vi "Handle Messages.vi"(8 "error in (no error)":errorcluster, 9 "Message Data":variant, 10 "Message":string, 11 "Process In":refnum<class "Debugger.lvclass">) -> (0 "error out":errorcluster, 3 "Process Out":refnum<class "Debugger.lvclass">)   [LabVIEW 2020, in "Debugger.lvclass"]
doc: "This is the core VI handling incomming messages to the process. This VI should be overridden to add functionality to the process or override functionality implemented by a parent. Any message not handled should be sent to the parent method using the default case. \nEach state should be atomic and states should in general avoid enqueueing new messages from within this method, as there might be other messages interleaved in the queue from the outside. For cyclic iteration of an action, using a Helper Loop is recommended."
uses:
  Debugger.lvclass
  C:/Users/anton/Documents/GitHub/triarc-debugger/source/Process/Debug Process.lvclass
  Debug Data/Debug Data.lvclass
  Debugger.lvclass/Debugger.ctl
  Debug Log/Debug Log.lvclass/Debug Log.ctl
  Process/Debug Process.lvclass/Debug Process.ctl
  State Analyzer/Debug State Analyzer.lvclass/Debug State Analyzer.ctl
  Process/Public/Lifecycle/Get Lifecycle State.vi
  <vilib>/Utility/error.llb/Clear Errors.vi
  <vilib>/Utility/error.llb/Error Cluster From Error Code.vi
  Process/Debug Process.lvclass
  Filter/Filter.lvclass
  Debug Log/Debug Log.lvclass
  State Analyzer/Debug State Analyzer.lvclass
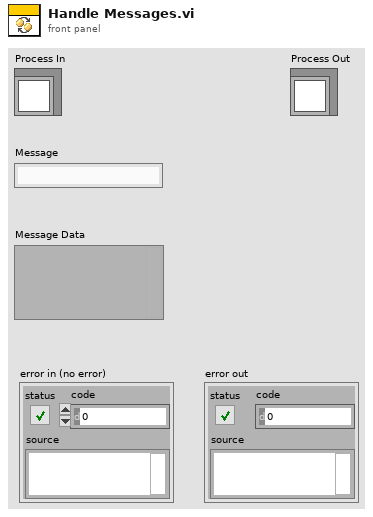
[diagram p1: front panel]
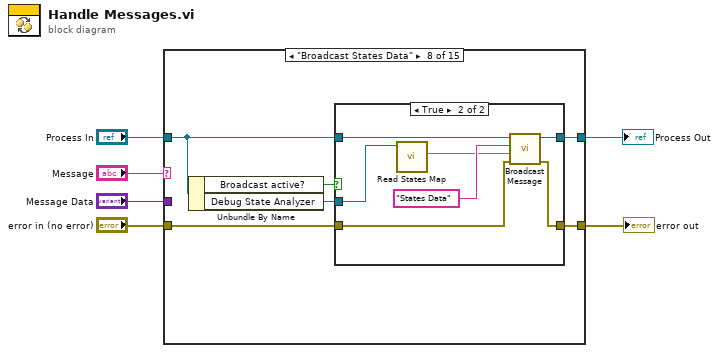
[diagram p0: block diagram]
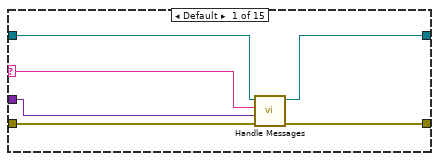
[diagram p2: hidden frame]
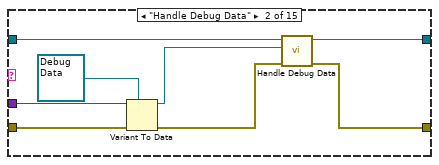
[diagram p3: hidden frame]
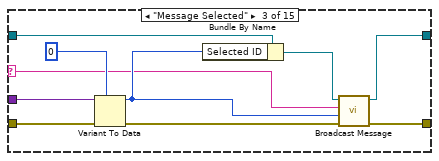
[diagram p4: hidden frame]
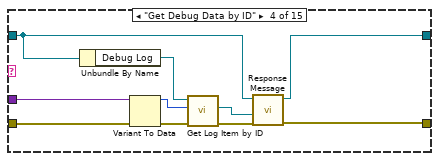
[diagram p5: hidden frame]
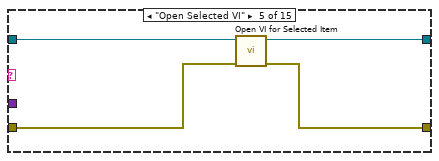
[diagram p6: hidden frame]
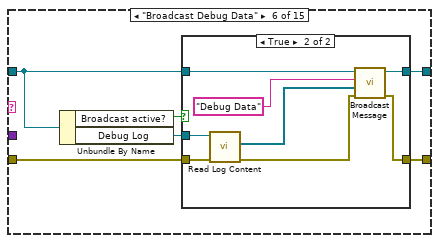
[diagram p7: hidden frame]
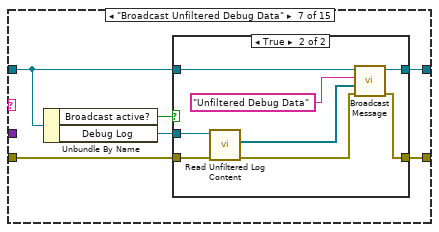
[diagram p9: hidden frame]
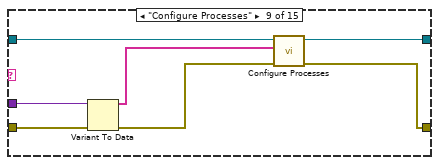
[diagram p12: hidden frame]
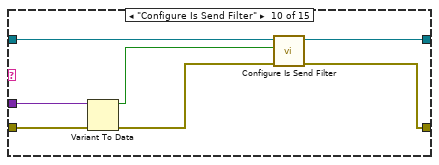
[diagram p13: hidden frame]
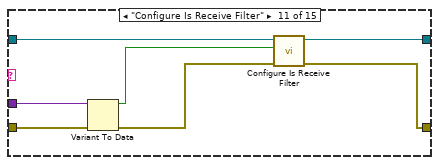
[diagram p14: hidden frame]
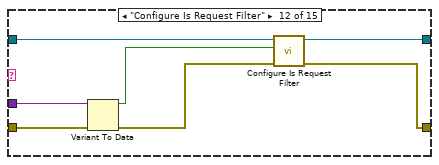
[diagram p15: hidden frame]
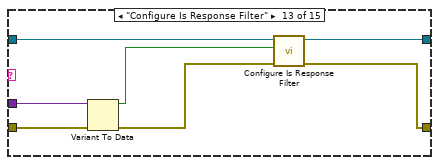
[diagram p16: hidden frame]
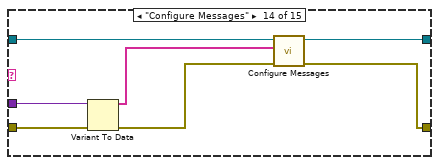
[diagram p17: hidden frame]
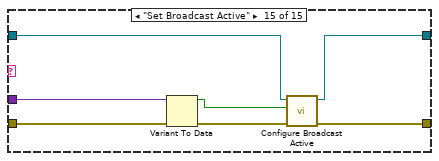
[diagram p18: hidden frame]
diagram:
  n1 = case shown="\"Broadcast States Data\"" "Message" {
    selector: "Message" -> [w8 _ w22 _ _ _ _ _ _ _ _ _ _ _ _]
    tunnel: [w12 w13 w25 w39 w41 w49 w65 w81 w93 w100 w107 w114 w121 w128 w137] -> w6
    tunnel: [w11 w15 w21 w40 w43 w50 w66 w82 w94 w101 w108 w115 w122 w129 w134] -> w5
    tunnel: "error in (no error)" -> [w10 w19 w29 w36 w44 w46 w62 w78 w98 w105 w112 w119 w126 w133 w139]
    tunnel: "Message Data" -> [w9 w20 w30 w37 _ _ _ _ w97 w104 w111 w118 w125 w132 w140]
    tunnel: "Process In" -> [w7 w16 w27 w32 w42 w48 w64 w80 w95 w102 w109 w116 w123 w130 w136]
    frame Default {
      n2 = call-parent "Handle Messages.vi"("error in (no error)"=w10, "Message Data"=w9, "Message"=w8, "Process In"=w7) -> ("error out"=w12:errorcluster, "Process Out"=w11:refnum<class "Debugger.lvclass">)  [unwired: 6 in]
    }
    frame "Handle Debug Data" {
      n3 = Variant To Data(error in=w19, type=refnum<class "Debug Data.lvclass"> refnum ("Debug Data.lvclass"), Variant=w20) -> (data=w14:refnum<class "Debug Data.lvclass">, error out=w17:errorcluster)
      n4 = call-dynamic "Handle Debug Data.vi"("error in (no error)"=w17, "Debug Data.lvclass"=w14, "Debug Data Event In"=w16) -> ("error out"=w13:errorcluster, "Debug Data Event Out"=w15:refnum<class "Debugger.lvclass">)  [unwired: 7 in]
    }
    frame "Message Selected" {
      n5 = Variant To Data(error in=w29, type=u32 0 ("Message ID"), Variant=w30) -> (data=w23:u32, error out=w26:errorcluster)
      n6 = Bundle By Name(cluster=w27, "Selected ID"=w23) -> (w24:refnum<class "Debugger.lvclass">)
      n7 = call-dynamic "Broadcast Message.vi"("error in (no error)"=w26, "Message Data"=w23, "Message"=w22, "Process In"=w24) -> ("error out"=w25:errorcluster, "Process Out"=w21:refnum<class "Debugger.lvclass">)  [unwired: 6 in]
    }
    frame "Get Debug Data by ID" {
      n8 = Unbundle By Name(w32) -> ("Debug Log"=w38:refnum<class "Debug Log.lvclass">)
      n9 = Variant To Data(error in=w36, Variant=w37) -> (data=w35:u32, error out=w34:errorcluster)  [unwired: 1 in]
      n10 = call "Get Log Item by ID.vi"("error in (no error)"=w34, "ID"=w35, "Debug Log In"=w38) -> ("error out"=w31:errorcluster, "Data Log"=w33:refnum<class "Debug Data.lvclass">)  [unwired: 6 in, 1 out]
      n11 = call "Response Message.vi"("error in (no error)"=w31, "Response Message Data"=w33, "Process In"=w32) -> ("error out"=w39:errorcluster, "Process Out"=w40:refnum<class "Debugger.lvclass">)  [unwired: 7 in]
    }
    frame "Open Selected VI" {
      n12 = call "Open VI for Selected Item.vi"("error in (no error)"=w44, "Debugger In"=w42) -> ("error out"=w41:errorcluster, "Debugger Out"=w43:refnum<class "Debugger.lvclass">)  [unwired: 8 in]
    }
    frame "Broadcast Debug Data" {
      n13 = Unbundle By Name(w48) -> ("Broadcast active?"=w45:bool, "Debug Log"=w47:refnum<class "Debug Log.lvclass">)
      n14 = case shown="True" w45 {
        tunnel: [w52 w60] -> w50
        tunnel: [w51 w59] -> w49
        tunnel: w48 -> [w52 w57]
        tunnel: w47 -> [_ w56]
        tunnel: w46 -> [w51 w54]
        frame False {
        }
        frame True {
          n15 = call "Read Log Content.vi"("error in (no error)"=w54, "Debug Log In"=w56) -> ("error out"=w55:errorcluster, "Data Log"=w53:refnum<class "Debug Data.lvclass">[])  [unwired: 7 in, 1 out]
          n16 = call-dynamic "Broadcast Message.vi"("error in (no error)"=w55, "Message Data"=w53, "Message"="Debug Data", "Process In"=w57) -> ("error out"=w59:errorcluster, "Process Out"=w60:refnum<class "Debugger.lvclass">)  [unwired: 6 in]
        }
      }
    }
    frame "Broadcast Unfiltered Debug Data" {
      n17 = Unbundle By Name(w64) -> ("Broadcast active?"=w61:bool, "Debug Log"=w63:refnum<class "Debug Log.lvclass">)
      n18 = case shown="True" w61 {
        tunnel: [w68 w76] -> w66
        tunnel: [w67 w75] -> w65
        tunnel: w64 -> [w68 w73]
        tunnel: w63 -> [_ w72]
        tunnel: w62 -> [w67 w70]
        frame False {
        }
        frame True {
          n19 = call "Read Unfiltered Log Content.vi"("error in (no error)"=w70, "Debug Log In"=w72) -> ("error out"=w71:errorcluster, "Data Log"=w69:refnum<class "Debug Data.lvclass">[])  [unwired: 7 in, 1 out]
          n20 = call-dynamic "Broadcast Message.vi"("error in (no error)"=w71, "Message Data"=w69, "Message"="Unfiltered Debug Data", "Process In"=w73) -> ("error out"=w75:errorcluster, "Process Out"=w76:refnum<class "Debugger.lvclass">)  [unwired: 6 in]
        }
      }
    }
    frame "Broadcast States Data" {
      n21 = Unbundle By Name(w80) -> ("Broadcast active?"=w77:bool, "Debug State Analyzer"=w79:refnum<class "Debug State Analyzer.lvclass">)
      n22 = case shown="True" w77 {
        tunnel: [w84 w91] -> w82
        tunnel: [w83 w90] -> w81
        tunnel: w80 -> [w84 w88]
        tunnel: w79 -> [_ w87]
        tunnel: w78 -> [w83 w86]
        frame False {
        }
        frame True {
          n23 = call "Read States Map.vi"("Debug State Analyzer in"=w87) -> ("State Map"=w85:map{string, string})  [unwired: 9 in, 1 out]
          n24 = call-dynamic "Broadcast Message.vi"("error in (no error)"=w86, "Message Data"=w85, "Message"="States Data", "Process In"=w88) -> ("error out"=w90:errorcluster, "Process Out"=w91:refnum<class "Debugger.lvclass">)  [unwired: 6 in]
        }
      }
    }
    frame "Configure Processes" {
      n25 = Variant To Data(error in=w98, Variant=w97) -> (data=w96:string[], error out=w92:errorcluster)  [unwired: 1 in]
      n26 = call "Configure Processes.vi"("error in (no error)"=w92, "Processes"=w96, "Debugger In"=w95) -> ("error out"=w93:errorcluster, "Debugger Out"=w94:refnum<class "Debugger.lvclass">)  [unwired: 7 in]
    }
    frame "Configure Is Send Filter" {
      n27 = Variant To Data(error in=w105, Variant=w104) -> (data=w103:bool, error out=w99:errorcluster)  [unwired: 1 in]
      n28 = call "Configure Is Send Filter.vi"("error in (no error)"=w99, "Show Send?"=w103, "Debugger In"=w102) -> ("error out"=w100:errorcluster, "Debugger Out"=w101:refnum<class "Debugger.lvclass">)  [unwired: 7 in]
    }
    frame "Configure Is Receive Filter" {
      n29 = Variant To Data(error in=w112, Variant=w111) -> (data=w110:bool, error out=w106:errorcluster)  [unwired: 1 in]
      n30 = call "Configure Is Receive Filter.vi"("error in (no error)"=w106, "Show Receive?"=w110, "Debugger In"=w109) -> ("error out"=w107:errorcluster, "Debugger Out"=w108:refnum<class "Debugger.lvclass">)  [unwired: 7 in]
    }
    frame "Configure Is Request Filter" {
      n31 = Variant To Data(error in=w119, Variant=w118) -> (data=w117:bool, error out=w113:errorcluster)  [unwired: 1 in]
      n32 = call "Configure Is Request Filter.vi"("error in (no error)"=w113, "Show Request?"=w117, "Debugger In"=w116) -> ("error out"=w114:errorcluster, "Debugger Out"=w115:refnum<class "Debugger.lvclass">)  [unwired: 7 in]
    }
    frame "Configure Is Response Filter" {
      n33 = Variant To Data(error in=w126, Variant=w125) -> (data=w124:bool, error out=w120:errorcluster)  [unwired: 1 in]
      n34 = call "Configure Is Response Filter.vi"("error in (no error)"=w120, "Show Response?"=w124, "Debugger In"=w123) -> ("error out"=w121:errorcluster, "Debugger Out"=w122:refnum<class "Debugger.lvclass">)  [unwired: 7 in]
    }
    frame "Configure Messages" {
      n35 = Variant To Data(error in=w133, Variant=w132) -> (data=w131:string[], error out=w127:errorcluster)  [unwired: 1 in]
      n36 = call "Configure Messages.vi"("error in (no error)"=w127, "Messages"=w131, "Debugger In"=w130) -> ("error out"=w128:errorcluster, "Debugger Out"=w129:refnum<class "Debugger.lvclass">)  [unwired: 7 in]
    }
    frame "Set Broadcast Active" {
      n37 = Variant To Data(error in=w139, Variant=w140) -> (data=w135:bool, error out=w138:errorcluster)  [unwired: 1 in]
      n38 = call "Configure Broadcast Active.vi"("error in (no error)"=w138, "Active?"=w135, "Debugger In"=w136) -> ("error out"=w137:errorcluster, "Debugger Out"=w134:refnum<class "Debugger.lvclass">)  [unwired: 7 in]
    }
  }
  "error out" <- w6
  "Process Out" <- w5
